vi "tra25cc_goto_z-absolute.vi"(8 "error in (no error)":errorcluster, 10 "z_val":dbl, 11 "conn_xyz_in":T2) -> (0 "error out":errorcluster, 3 "conn_xyz_out":T1)   [LabVIEW 2014]
uses:
  D:/Microscope/Software/Tools/Stage_xyz/Dll/Newport.CONEXCC.CommandInterface.dll
  Tools/Stage_xyz/Dll/Newport.CONEXCC.CommandInterface.dll
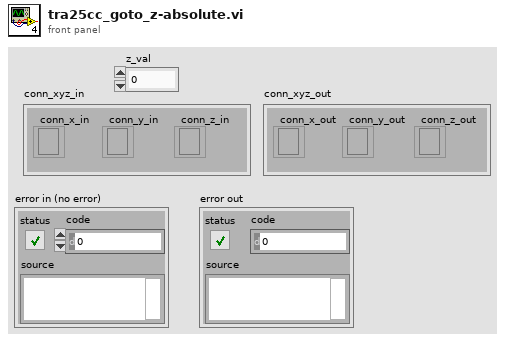
[diagram p1: front panel]
types:
  T1 = cluster{"conn_x_out":refnum<k24>, "conn_y_out":refnum<k24>, "conn_z_out":refnum<k24>}
  T2 = cluster{"conn_x_in":refnum<k24>, "conn_y_in":refnum<k24>, "conn_z_in":refnum<k24>}
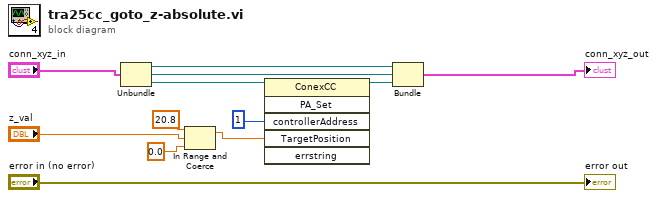
[diagram p0: block diagram]
diagram:
  n1 = Unbundle("conn_xyz_in") -> ("conn_x_in"=w4:refnum<k24>, "conn_y_in"=w3:refnum<k24>, "conn_z_in"=w6:refnum<k24>)
  n2 = In Range and Coerce(upper limit=20.8, x="z_val", lower limit=0.0) -> (coerced(x)=w1:dbl)  [unwired: 1 out]
  n3 = invoke class="ConexCC" method="PA_Set"(reference=w6, "controllerAddress"=1, "TargetPosition"=w1) -> (reference out=w5:refnum<k24>)  [unwired: 3 in, 5 out]
  n4 = Bundle("conn_x_in"=w4, "conn_y_in"=w3, "conn_z_in"=w5) -> (→"conn_xyz_out":T2)  [unwired: 1 in]
  "error out" <- "error in (no error)"
